vi "CS-4 Get Switch Heater.vi"(0 "VISA session":refnum<visa-resource-name>, 1 "error in (no error)":errorcluster) -> (2 "dup VISA session":refnum<visa-resource-name>, 4 "switch heater":bool, 5 "error out":errorcluster)   [LabVIEW 2020]
doc: "CS-4 Get Switch Heater.vi will return the switch heater status as a boolean."
panel:
  # "On"
  # "Off"
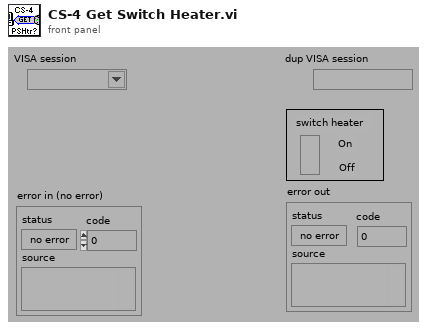
[diagram p1: front panel]
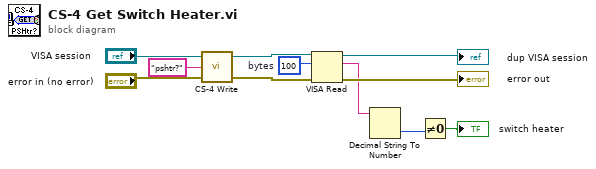
[diagram p0: block diagram]
diagram:
  w5 = u32 100  # bytes
  n1 = call "CS-4 Write.vi"("error in (no error)"="error in (no error)", "write buffer (\"\")"="pshtr?", "VISA session"="VISA session") -> ("error out"=w8:errorcluster, "dup VISA session"=w9:refnum<visa-resource-name>)  [unwired: 1 out]
  n2 = VISA Read(VISA resource name=w9, byte count=w5, error in (no error)=w8) -> (VISA resource name out=→"dup VISA session":refnum<visa-resource-name>, read buffer=w3:string, error out=→"error out":errorcluster)  [unwired: 1 out]
  n3 = Decimal String To Number(string=w3) -> (number=w2:i32)  [unwired: 2 in, 1 out]
  n4 = Not Equal To 0?(x=w2) -> (x != 0?=→"switch heater":bool)
